vi "McPhersonStateMachine.vi"   [LabVIEW 2020]
types:
  T1 = enum16{"_Quit_", "Idle", "Get Z0", "Get Status", "Slew to Z1", "Move@V", "Stop"}
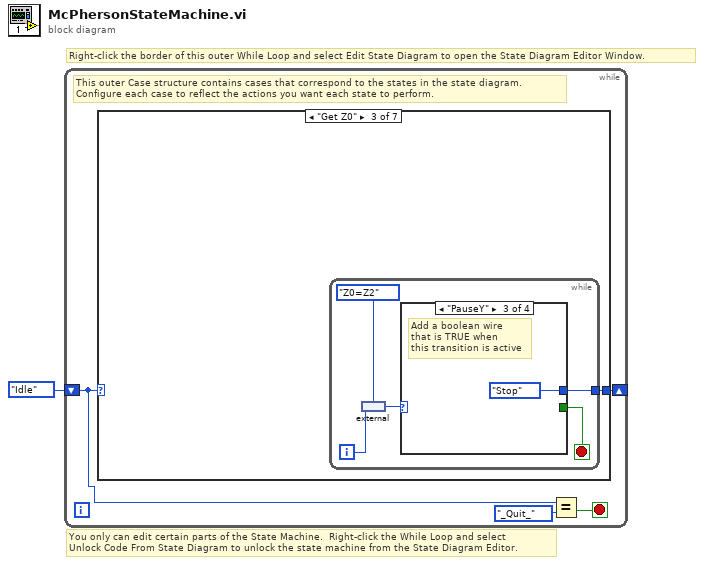
[diagram p0: block diagram]
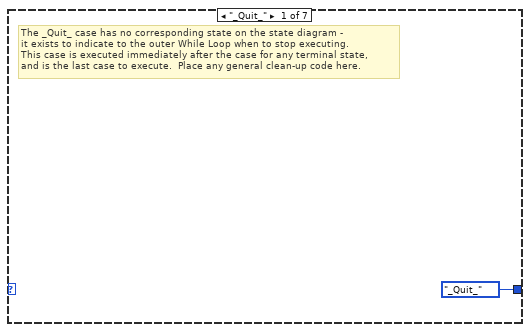
[diagram p2: hidden frame]
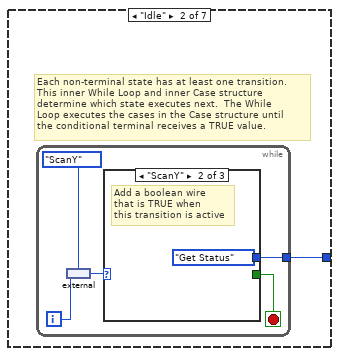
[diagram p3: hidden frame]
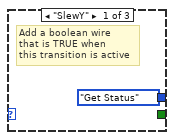
[diagram p4: hidden frame]
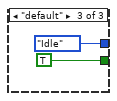
[diagram p5: hidden frame]
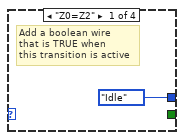
[diagram p6: hidden frame]
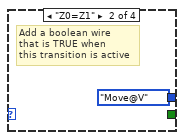
[diagram p7: hidden frame]
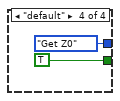
[diagram p8: hidden frame]
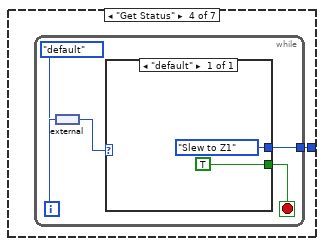
[diagram p9: hidden frame]
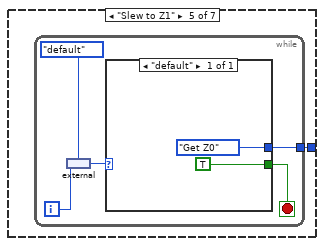
[diagram p10: hidden frame]
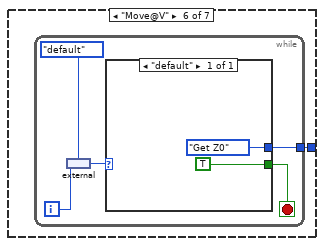
[diagram p11: hidden frame]
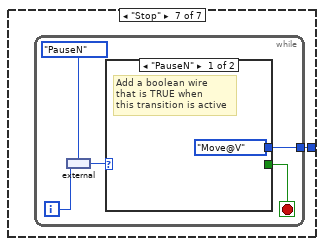
[diagram p12: hidden frame]
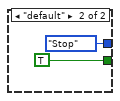
[diagram p13: hidden frame]
diagram:
  # "Right-click the border of this outer While Loop and select Edit State Diagram to open the State Diagram Editor Window."
  # "You only can edit certain parts of the State Machine.  Right-click the While Loop and select \nUnlock Code From State Diagram to unlock the state machine from the State Diagram Editor."
  n1 = while {
    shift-right: [w4] -> _
    shift-left: T1."Idle" -> [w5]
    stop <- w3 stop-if-true
    # "This outer Case structure contains cases that correspond to the states in the state diagram.  \nConfigure each case to reflect the actions you want each state to perform."
    n2 = case shown="\"Get Z0\"" w5 {
      tunnel: [T1."_Quit_" w7 w22 w38 w51 w64 w77] -> w4
      frame "_Quit_" {
        # "The _Quit_ case has no corresponding state on the state diagram -\nit exists to indicate to the outer While Loop when to stop executing.\nThis case is executed immediately after the case for any terminal state, \nand is the last case to execute.  Place any general clean-up code here."
      }
      frame "Idle" {
        # "Each non-terminal state has at least one transition.\nThis inner While Loop and inner Case structure \ndetermine which state executes next.  The While \nLoop executes the cases in the Case structure until \nthe conditional terminal receives a TRUE value."
        n3 = while {
          tunnel: [w9] -> w7
          i -> [w12]
          stop <- w8 stop-if-true
          n4 = external(enum16{"SlewY", "ScanY", "default"}."ScanY", w12) -> (w10:enum16{"SlewY", "ScanY", "default"})
          n5 = case shown="\"ScanY\"" w10 {
            tunnel: [T1."Get Status" T1."Get Status" T1."Idle"] -> w9
            tunnel: [_ _ TRUE] -> w8
            frame "SlewY" {
              # "Add a boolean wire\nthat is TRUE when\nthis transition is active"
            }
            frame "ScanY" {
              # "Add a boolean wire\nthat is TRUE when\nthis transition is active"
            }
            frame "default" {
            }
          }
        }
      }
      frame "Get Z0" {
        n6 = while {
          tunnel: [w24] -> w22
          i -> [w27]
          stop <- w23 stop-if-true
          n7 = external(enum16{"Z0=Z2", "Z0=Z1", "PauseY", "default"}."Z0=Z2", w27) -> (w25:enum16{"Z0=Z2", "Z0=Z1", "PauseY", "default"})
          n8 = case shown="\"PauseY\"" w25 {
            tunnel: [T1."Idle" T1."Move@V" T1."Stop" T1."Get Z0"] -> w24
            tunnel: [_ _ _ TRUE] -> w23
            frame "Z0=Z2" {
              # "Add a boolean wire\nthat is TRUE when\nthis transition is active"
            }
            frame "Z0=Z1" {
              # "Add a boolean wire\nthat is TRUE when\nthis transition is active"
            }
            frame "PauseY" {
              # "Add a boolean wire\nthat is TRUE when\nthis transition is active"
            }
            frame "default" {
            }
          }
        }
      }
      frame "Get Status" {
        n9 = while {
          tunnel: [w41] -> w38
          i -> [w43]
          stop <- w40 stop-if-true
          n10 = external(enum16{"default"}."default", w43) -> (w42:enum16{"default"})
          n11 = case shown="\"default\"" w42 {
            tunnel: [T1."Slew to Z1"] -> w41
            tunnel: [TRUE] -> w40
            frame "default" {
            }
          }
        }
      }
      frame "Slew to Z1" {
        n12 = while {
          tunnel: [w53] -> w51
          i -> [w56]
          stop <- w52 stop-if-true
          n13 = external(enum16{"default"}."default", w56) -> (w54:enum16{"default"})
          n14 = case shown="\"default\"" w54 {
            tunnel: [T1."Get Z0"] -> w53
            tunnel: [TRUE] -> w52
            frame "default" {
            }
          }
        }
      }
      frame "Move@V" {
        n15 = while {
          tunnel: [w66] -> w64
          i -> [w69]
          stop <- w65 stop-if-true
          n16 = external(enum16{"default"}."default", w69) -> (w67:enum16{"default"})
          n17 = case shown="\"default\"" w67 {
            tunnel: [T1."Get Z0"] -> w66
            tunnel: [TRUE] -> w65
            frame "default" {
            }
          }
        }
      }
      frame "Stop" {
        n18 = while {
          tunnel: [w79] -> w77
          i -> [w82]
          stop <- w78 stop-if-true
          n19 = external(enum16{"PauseN", "default"}."PauseN", w82) -> (w80:enum16{"PauseN", "default"})
          n20 = case shown="\"PauseN\"" w80 {
            tunnel: [T1."Move@V" T1."Stop"] -> w79
            tunnel: [_ TRUE] -> w78
            frame "PauseN" {
              # "Add a boolean wire\nthat is TRUE when\nthis transition is active"
            }
            frame "default" {
            }
          }
        }
      }
    }
    n21 = Equal?(x=w5, y=T1."_Quit_") -> (x = y?=w3:bool)
  }
